vi "FTW-Request-AddMetaData.vi"(0 "Response":refnum<data-value>, 5 "Include Exception":bool=TRUE, 7 "Include Timestamp":bool, 9 "Include Relative Timer":bool, 11 "error in":errorcluster) -> (4 "Response out":refnum<data-value>, 15 "error out":errorcluster)   [LabVIEW 2015]
doc: "Sends a response message back to the requesting client. This message is attempts to send unconditionally of incoming error. Take caution to wire a sanitized error into this function, because it will be repeated back onto the client. Said another way, an error generated while processing the request will be not only thrown on the request handler, but also on the client as well."
uses:
  json/core/FTW-JSON-Core-Structure.ctl
  time/FTW-Time-DisplayFormat-Timestamp.ctl
panel:
  # "Inputs"
  # "Outputs"
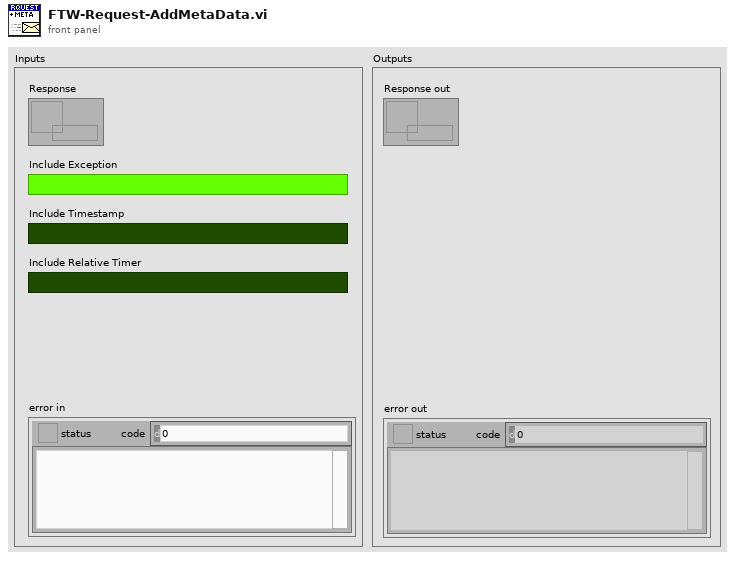
[diagram p1: front panel]
types:
  T1 = typedef "FTW-ERR-ExceptionType.ctl" = enum16{"OK", "Info", "Warning", "Error"}
  T2 = typedef "FTW-Time-DisplayFormat-Timestamp.ctl" = enum16{"YYYY-MM-DDT00:00:00.000Z (ISO-8601)", "YYYY-MM-DDT00-00-00Z (Simple ISO-8601)", "YYYY-MM-DD"}
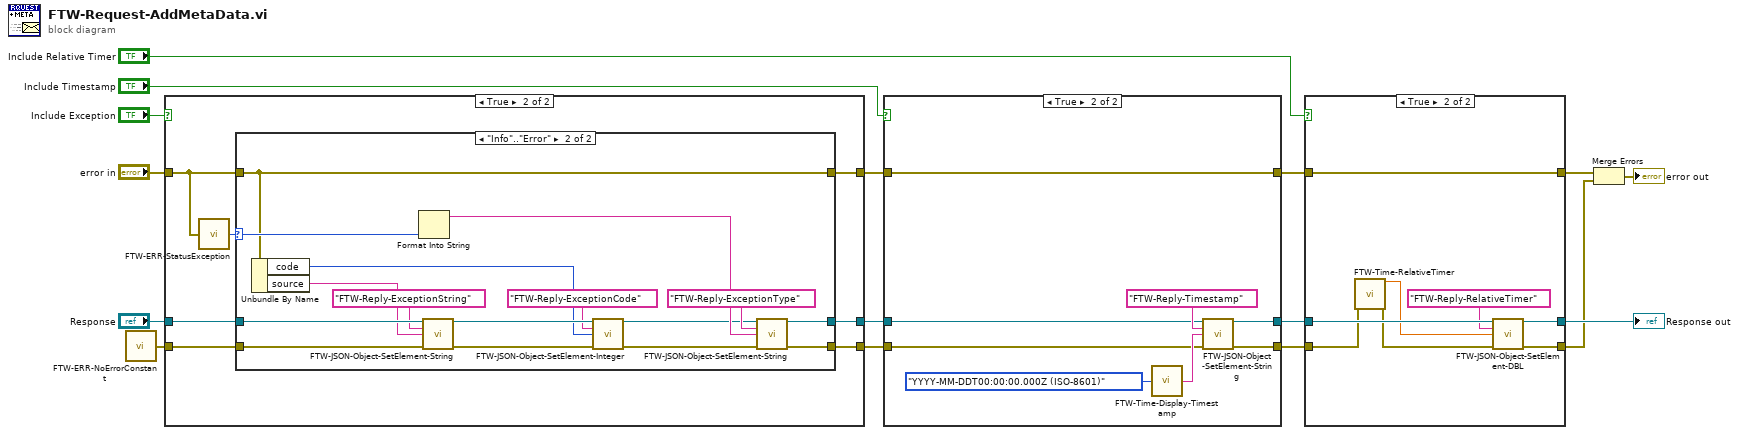
[diagram p0: block diagram]
diagram:
  n1 = call "FTW-ERR-NoErrorConstant.vi"() -> ("no error"=w8:errorcluster)
  n2 = case shown="True" "Include Exception" {
    tunnel: [w18 w25] -> w9
    tunnel: [w19 w24] -> w4
    tunnel: "Response" -> [w18 w23]
    tunnel: "error in" -> [w19 w22]
    tunnel: w8 -> [w17 w21]
    tunnel: [w17 w20] -> w7
    frame False {
    }
    frame True {
      n3 = call "FTW-ERR-StatusException.vi"("error to check"=w22) -> ("Exception"=w26:T1)
      n4 = case shown="\"Info\"..\"Error\"" w26 {
        selector: w26 -> [_ w43]
        tunnel: w23 -> [w29 w45]
        tunnel: [w29 w42] -> w25
        tunnel: w22 -> [w28 w31]
        tunnel: [w28 w31] -> w24
        tunnel: w21 -> [w27 w32]
        tunnel: [w27 w30] -> w20
        frame "OK" {
        }
        frame "Info".."Error" {
          n5 = Unbundle By Name(w31) -> ("code"=w37:i32, "source"=w35:string)
          n6 = Format Into String(w43) -> (resulting string=w40:string)  [unwired: 3 in, 1 out]
          n7 = call "FTW-JSON-Object-SetElement-String.vi"("JSON Object"=w45, "Key"="FTW-Reply-ExceptionString", "Value"=w35, "error in"=w32) -> ("JSON Object out"=w39:refnum<data-value>, "error out"=w34:errorcluster)  [unwired: 10 in]
          n8 = call "FTW-JSON-Object-SetElement-Integer.vi"("JSON Object"=w39, "Key"="FTW-Reply-ExceptionCode", "Value"=w37, "error in"=w34) -> ("JSON Object out"=w38:refnum<data-value>, "error out"=w33:errorcluster)  [unwired: 10 in]
          n9 = call "FTW-JSON-Object-SetElement-String.vi"("JSON Object"=w38, "Key"="FTW-Reply-ExceptionType", "Value"=w40, "error in"=w33) -> ("JSON Object out"=w42:refnum<data-value>, "error out"=w30:errorcluster)  [unwired: 10 in]
        }
      }
    }
  }
  n10 = case shown="True" "Include Timestamp" {
    tunnel: [w47 w53] -> w16
    tunnel: [w46 w52] -> w3
    tunnel: w9 -> [w47 w51]
    tunnel: w7 -> [w46 w50]
    tunnel: [w48 w49] -> w5
    tunnel: w4 -> [w48 w49]
    frame False {
    }
    frame True {
      n11 = call "FTW-Time-Display-Timestamp.vi"("Format"=FTW-Time-DisplayFormat-Timestamp."YYYY-MM-DDT00:00:00.000Z (ISO-8601)") -> ("Formatted Timestamp"=w54:string)  [unwired: 3 in]
      n12 = call "FTW-JSON-Object-SetElement-String.vi"("JSON Object"=w51, "Key"="FTW-Reply-Timestamp", "Value"=w54, "error in"=w50) -> ("JSON Object out"=w53:refnum<data-value>, "error out"=w52:errorcluster)  [unwired: 10 in]
    }
  }
  n13 = case shown="True" "Include Relative Timer" {
    tunnel: w16 -> [w59 w67]
    tunnel: w3 -> [w57 w65]
    tunnel: [w59 w62] -> w12
    tunnel: [w58 w60] -> w6
    tunnel: w5 -> [w58 w60]
    tunnel: [w57 w61] -> w2
    frame False {
    }
    frame True {
      n14 = call "FTW-Time-RelativeTimer.vi"("error in"=w65) -> ("Current Timer Value"=w63:dbl, "error out"=w64:errorcluster)  [unwired: 12 in, 1 out]
      n15 = call "FTW-JSON-Object-SetElement-DBL.vi"("JSON Object"=w67, "Key"="FTW-Reply-RelativeTimer", "Value"=w63, "error in"=w64) -> ("JSON Object out"=w62:refnum<data-value>, "error out"=w61:errorcluster)  [unwired: 10 in]
    }
  }
  "Response out" <- w12
  n16 = Merge Errors(w6, w2) -> (→"error out":errorcluster)
